vi "origin.vi"(8 "error in (no error)":errorcluster, 11 "vi ref":refnum<vi>) -> (0 "error out":errorcluster, 3 "vi ref":refnum<vi>)   [LabVIEW 2021, in "Autocomplete popup.lvlib"]
uses:
  Autocomplete popup.lvlib
  <vilib>/Utility/miscctls.llb/LVPointTypeDef.ctl
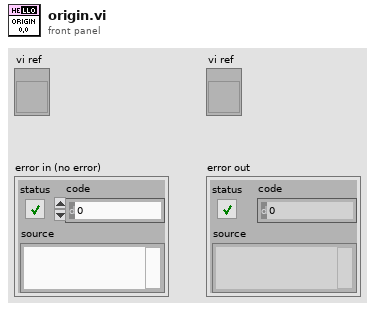
[diagram p1: front panel]
types:
  T1 = typedef "LVPointTypeDef.ctl" = cluster{"Horizontal":i16, "Vertical":i16}
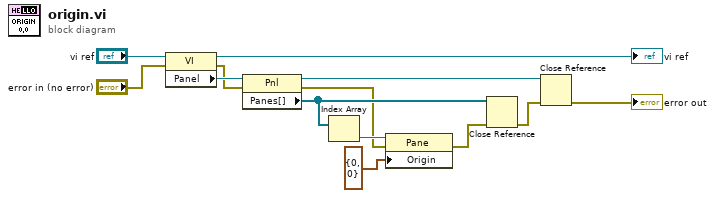
[diagram p0: block diagram]
diagram:
  n1 = property class="VI"(reference="vi ref", error in="error in (no error)") -> (reference out=→"vi ref":refnum<vi>, error out=w9:errorcluster, "Panel"=w13:refnum<vi>)
  n2 = property class="Pnl"(reference=w13, error in=w9) -> (reference out=w7:refnum<vi>, error out=w5:errorcluster, "Panes[]"=w10:refnum<vi>[])
  n3 = Index Array(array=w10) -> (element=w11:refnum<vi>)  [unwired: 1 in]
  n4 = property class="Pane"(reference=w11, error in=w5, "Origin"=T1 {"Horizontal"=0, "Vertical"=0}) -> (error out=w8:errorcluster)  [unwired: 1 out]
  n5 = Close Reference(reference=w10, error in (no error)=w8) -> (error out=w6:errorcluster)
  n6 = Close Reference(reference=w7, error in (no error)=w6) -> (error out=→"error out":errorcluster)
